vi "Actualizar Cafes.vi"(11 "Cluster Producto":T1) -> ()   [LabVIEW 2019, in "CAFE ACTOR.lvlib" / "CAFE ACTOR.lvclass"]
uses:
  CAFE ACTOR.lvclass
  <vilib>/Utility/config.llb/Write Key (I32).vi
  <vilib>/Utility/config.llb/NI_LVConfig.lvlib
panel:
  in  "CAFE ACTOR in":refnum<class "CAFE ACTOR.lvclass">
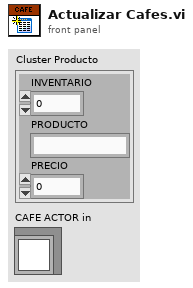
[diagram p1: front panel]
types:
  T1 = cluster{"INVENTARIO":i32, "PRODUCTO":string, "PRECIO":dbl}
  T2 = typedef "NI_LVConfig.lvlib/Config Data RefNum.ctl" = refnum<k1>
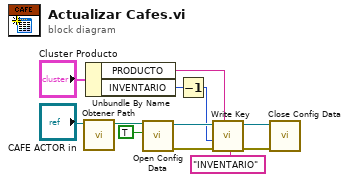
[diagram p0: block diagram]
diagram:
  n1 = call "Obtener Path.vi"("CAFE ACTOR.lvlib:CAFE ACTOR.lvclass"="CAFE ACTOR in") -> ("appended path"=w2:path)  [unwired: 10 in]
  n2 = Unbundle By Name("Cluster Producto") -> ("PRODUCTO"=w5:string, "INVENTARIO"=w4:i32)
  n3 = call <vilib>:"Open Config Data.vi"("create file if necessary (T)"=TRUE, "configuration file path"=w2) -> ("error out"=w10:errorcluster, "refnum"=w11:T2)  [unwired: 7 in, 1 out]
  n4 = Decrement(x=w4) -> (x-1=w3:i32)
  n5 = call-poly <vilib>:"Write Key.vi"("section"=w5, "error in (no error)"=w10, "value"=w3, "key"="INVENTARIO", "refnum"=w11) -> ("error out"=w9:errorcluster, "refnum out"=w8:T2)  [unwired: 4 in, 1 out]
  n6 = call <vilib>:"Close Config Data.vi"("error in (no error)"=w9, "refnum"=w8) -> ()  [unwired: 8 in, 2 out]
